vi "Telnet Buffered Read.vi"(7 "unfiltered buffer in":string, 8 "error in (no error)":errorcluster, 9 "read info":T1={"bytes to read"=60, "timeout ms"=100, "read mode"=enum."normal", "line separator"="login: "}, 10 "buffer in":string, 11 "connection ID":refnum<k5>) -> (0 "error out":errorcluster, 1 "data":string, 2 "buffer out":string, 3 "connection ID out":refnum<k5>, 4 "unfiltered buffer out":string)   [LabVIEW 2015, in "NI_InternetTK_Core_VIs.lvlib"]
uses:
  NI_InternetTK_Core_VIs.lvlib
  NI_InternetTK_Common_VIs.lvlib
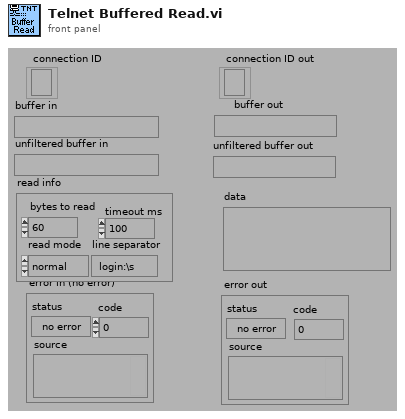
[diagram p1: front panel]
types:
  T1 = cluster{"bytes to read":i32, "timeout ms":i32, "read mode":enum16{"normal", "line", "buffered"}, "line separator":string}
  T2 = enum16{"Standard", "Buffered", "CRLF", "Immediate"}
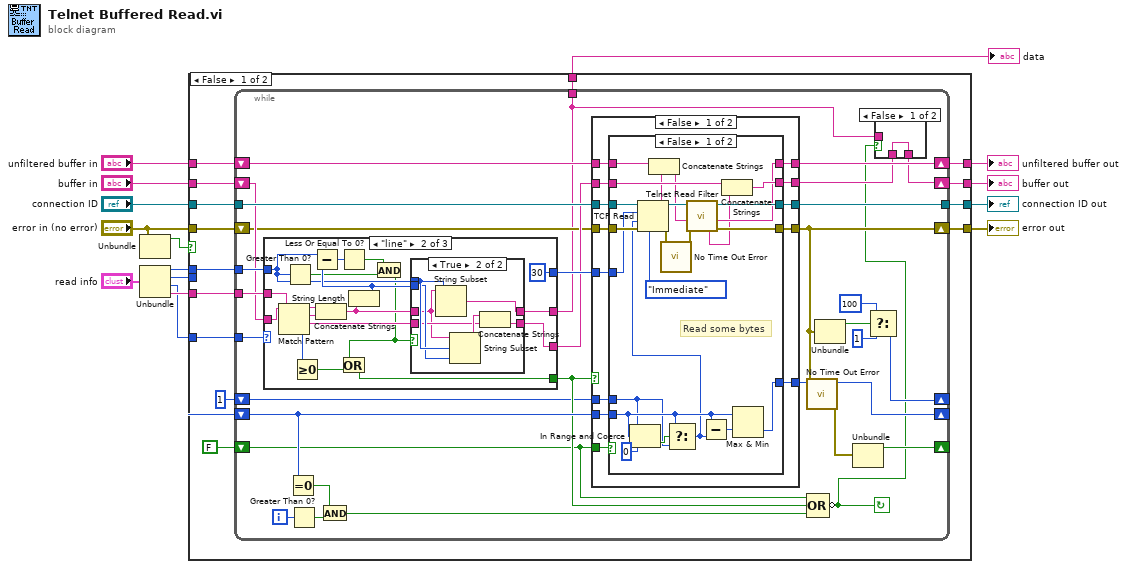
[diagram p0: block diagram]
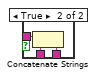
[diagram p2: hidden frame]
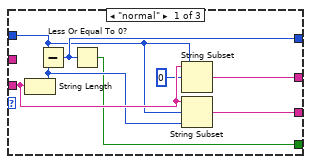
[diagram p3: hidden frame]
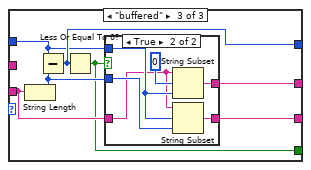
[diagram p5: hidden frame]
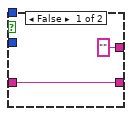
[diagram p6: hidden frame]
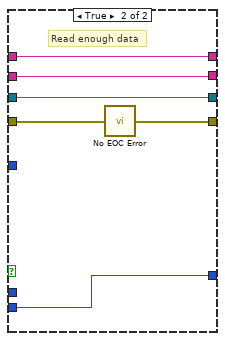
[diagram p8: hidden frame]
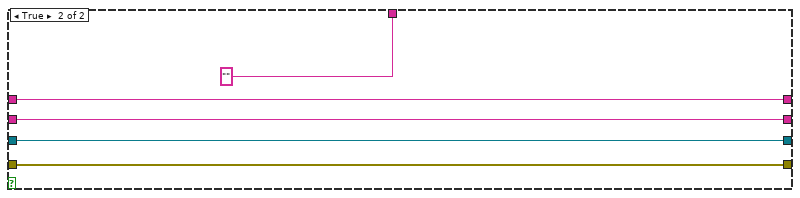
[diagram p9: hidden frame]
diagram:
  n1 = Unbundle("error in (no error)") -> ("status"=w3:bool)  [unwired: 2 out]
  n2 = Unbundle("read info") -> ("bytes to read"=w13:i32, "timeout ms"=w12:i32, "read mode"=w5:enum16{"normal", "line", "buffered"}, "line separator"=w11:string)
  n3 = case shown="False" w3 {
    tunnel: "buffer in" -> [w30 w165]
    tunnel: w13 -> [w19 _]
    tunnel: w12 -> [w27 _]
    tunnel: "connection ID" -> [w28 w164]
    tunnel: w11 -> [w29 _]
    tunnel: "error in (no error)" -> [w17 w167]
    tunnel: [w26 w164] -> w9
    tunnel: [w16 w167] -> w8
    tunnel: [w25 w165] -> w2
    tunnel: "unfiltered buffer in" -> [w23 w166]
    tunnel: [w22 w166] -> w6
    tunnel: w5 -> [w20 _]
    tunnel: [w18 "" ("substring")] -> w1
    frame False {
      n4 = while {
        shift-left: w17 -> [w36]
        shift-right: [w35] -> w16
        tunnel: [w31] -> w18
        tunnel: w19 -> [w39]
        tunnel: w20 -> [w40]
        shift-left: 1 ("bytes to read") -> [w46]
        shift-right: [w42] -> _
        shift-left: w23 -> [w50]
        shift-right: [w49] -> w22
        shift-left: FALSE ("status") -> [w51]
        shift-right: [w47] -> _
        tunnel: [w58] -> w26
        shift-left: w27 -> [w57]
        shift-right: [w59] -> _
        tunnel: w28 -> [w60]
        tunnel: w29 -> [w61]
        shift-left: w30 -> [w38]
        shift-right: [w33] -> w25
        i -> [w56]
        stop <- w32 continue-if-true
        n5 = case shown="\"line\"" w40 {
          tunnel: [w68 30 ("bytes to read") w102] -> w41
          tunnel: [w72 w80 w106] -> w31
          tunnel: [w69 w83 w103] -> w52
          tunnel: w38 -> [w73 w89 w107]
          tunnel: [w70 w79 w104] -> w37
          tunnel: w61 -> [_ w87 _]
          tunnel: w39 -> [w66 w77 w101]
          frame "normal" {
            n6 = String Length(string=w73) -> (length=w71:i32)
            n7 = Subtract(x=w66, y=w71) -> (x-y=w68:i32)
            n8 = Less Or Equal To 0?(x=w68) -> (x <= 0?=w69:bool)
            n9 = String Subset(string=w73, offset (0)=0 ("length"), length (rest)=w66) -> (substring=w72:string)
            n10 = String Subset(string=w73, offset (0)=w66, length (rest)=w71) -> (substring=w70:string)
          }
          frame "line" {
            n11 = Match Pattern(string=w89, regular expression=w87) -> (before substring=w88:string, match substring=w90:string, after substring=w81:string, offset past match=w86:i32)  [unwired: 1 out]
            n12 = Greater Than 0?(x=w77) -> (x > 0?=w74:bool)
            n13 = Greater Or Equal To 0?(x=w86) -> (x >= 0?=w84:bool)
            n14 = Concatenate Strings(w88, w90) -> (w82:string)
            n15 = String Length(string=w82) -> (length=w78:i32)
            n16 = Subtract(x=w77, y=w78) -> (x-y=w85:i32)
            n17 = Less Or Equal To 0?(x=w85) -> (x <= 0?=w75:bool)
            n18 = And(x=w75, y=w74) -> (x .and. y?=w76:bool)
            n19 = Or(x=w76, y=w84) -> (x .or. y?=w83:bool)
            n20 = case shown="True" w76 {
              tunnel: w82 -> [w93 w94]
              tunnel: w81 -> [w92 w96]
              tunnel: [w93 w100] -> w80
              tunnel: [w92 w95] -> w79
              tunnel: w77 -> [_ w99]
              tunnel: w78 -> [_ w98]
              frame False {
              }
              frame True {
                n21 = String Subset(string=w94, length (rest)=w99) -> (substring=w100:string)  [unwired: 1 out]
                n22 = String Subset(string=w94, offset (0)=w99, length (rest)=w98) -> (substring=w97:string)
                n23 = Concatenate Strings(w97, w96) -> (w95:string)
              }
            }
          }
          frame "buffered" {
            n24 = String Length(string=w107) -> (length=w105:i32)
            n25 = Subtract(x=w101, y=w105) -> (x-y=w102:i32)
            n26 = Less Or Equal To 0?(x=w102) -> (x <= 0?=w103:bool)
            n27 = case shown="True" w103 {
              tunnel: [w109 w115] -> w104
              tunnel: w105 -> [_ w114]
              tunnel: ["" ("substring") w113] -> w106
              tunnel: w107 -> [w109 w110]
              tunnel: w101 -> [_ w112]
              frame False {
              }
              frame True {
                n28 = String Subset(string=w110, offset (0)=0 ("length"), length (rest)=w112) -> (substring=w113:string)
                n29 = String Subset(string=w110, offset (0)=w112, length (rest)=w114) -> (substring=w115:string)
              }
            }
          }
        }
        n30 = Equal To 0?(x=w57) -> (x = 0?=w55:bool)
        n31 = Greater Than 0?(x=w56) -> (x > 0?=w54:bool)
        n32 = And(x=w55, y=w54) -> (x .and. y?=w53:bool)
        n33 = case shown="False" w52 {
          tunnel: [w126 w157] -> w34
          tunnel: w37 -> [w128 w157]
          tunnel: [w120 w160] -> w35
          tunnel: w60 -> [w127 w161]
          tunnel: w57 -> [w124 w162]
          tunnel: [w123 w162] -> w59
          tunnel: [w125 w161] -> w58
          tunnel: w51 -> [w122 _]
          tunnel: w36 -> [w121 w159]
          tunnel: w50 -> [w119 w158]
          tunnel: [w118 w158] -> w49
          tunnel: w46 -> [w117 _]
          tunnel: w41 -> [w116 _]
          frame False {
            n34 = case shown="False" w122 {
              tunnel: [w151 w155] -> w123
              tunnel: w124 -> [w150 w155]
              tunnel: [w145 w156] -> w125
              tunnel: [w138 w152] -> w126
              tunnel: [w142 w154] -> w120
              tunnel: w127 -> [w146 w156]
              tunnel: w128 -> [w139 w152]
              tunnel: w121 -> [w144 w154]
              tunnel: w119 -> [w135 w153]
              tunnel: [w134 w153] -> w118
              tunnel: w117 -> [w133 _]
              tunnel: w116 -> [w132 _]
              frame False {
                # "Read some bytes"
                n35 = In Range and Coerce(upper limit=w133, x=w150, lower limit=0 ("bytes to read")) -> (In Range?=w148:bool)  [unwired: 1 out]
                n36 = Select(t=w150, s=w148, f=w133) -> (s? t:f=w131:i32)
                n37 = TCP Read(connection ID=w146, bytes to read=w132, error in (no error)=w144, 7:T2."Immediate" ("mode (standard)"), 9:w131) -> (connection ID out=w143:refnum<k5>, data out=w137:string, error out=w141:errorcluster)
                n38 = Concatenate Strings(w135, w137) -> (w136:string)
                n39 = call "No Time Out Error.vi"("error in (no error)"=w141) -> ("error out"=w140:errorcluster)  [unwired: 14 out]
                n40 = call "Telnet Read Filter.vi"("error in"=w140, "unfiltered data in"=w136, "Connection in"=w143) -> ("error out"=w142:errorcluster, "Unfiltered data out"=w134:string, "Data out"=w130:string, "connection out"=w145:refnum<k5>)  [unwired: 1 out]
                n41 = Subtract(x=w150, y=w131) -> (x-y=w149:i32)
                n42 = Concatenate Strings(w139, w130) -> (w138:string)
                n43 = Max & Min(x=w150, y=w149) -> (min(x,y)=w151:i32)  [unwired: 1 out]
              }
              frame True {
                # "Error! (Connection closed, etc.)"
              }
            }
          }
          frame True {
            # "Read enough data"
            n44 = call "No EOC Error.vi"("error in (no error)"=w159) -> ("error out"=w160:errorcluster)  [unwired: 4 out]
          }
        }
        n45 = call "No Time Out Error.vi"("error in (no error)"=w35) -> ("error out"=w48:errorcluster)  [unwired: 14 out]
        n46 = Compound Arithmetic op=OR(w51, w52, w53) -> (invert w32:bool)
        n47 = Unbundle(w35) -> ("status"=w45:bool)  [unwired: 2 out]
        n48 = Unbundle(w48) -> ("status"=w47:bool)  [unwired: 2 out]
        n49 = Select(t=100 ("bytes to read"), s=w45, f=1 ("bytes to read")) -> (s? t:f=w42:i32)
        n50 = case shown="False" w32 {
          tunnel: w34 -> [w62 w65]
          tunnel: [w62 w64] -> w33
          tunnel: w31 -> [_ w63]
          frame False {
          }
          frame True {
            n51 = Concatenate Strings(w63, w65) -> (w64:string)
          }
        }
      }
    }
    frame True {
    }
  }
  "error out" <- w8
  "connection ID out" <- w9
  "buffer out" <- w2
  "data" <- w1
  "unfiltered buffer out" <- w6
